vi "Scan Setup.vi"(8 "error in (no error)":errorcluster, 11 "Wavelength in":refnum<class "Wavelength Triax 550.lvclass">) -> (0 "error out":errorcluster, 3 "Wavelength out":refnum<class "Wavelength Triax 550.lvclass">)   [LabVIEW 2017, in "Wavelength Triax 550.lvclass"]
doc: "Configure the instrument based on the class member data. This step comes after the user has closed the \"Scan Setup\" window and before the actual scan -- so instruments are configured with the user's specified settings."
uses:
  Wavelength Triax 550.lvclass
  Instruments/Spectrometer Triax 550/JY-SPEX-TRIAX/controls.llb/Slits.ctl
  Wavelength Triax 550.lvclass/Wavelength Triax 550.ctl
  Scanner/Scanner.lvclass
  Instruments/Utility Classes/Scannable/Scannable.lvclass
  Instruments/Spectrometer Triax 550/JY-SPEX-TRIAX/JY-SPEX-TRIAX.lvlib
panel:
  out "User Cancelled?":bool
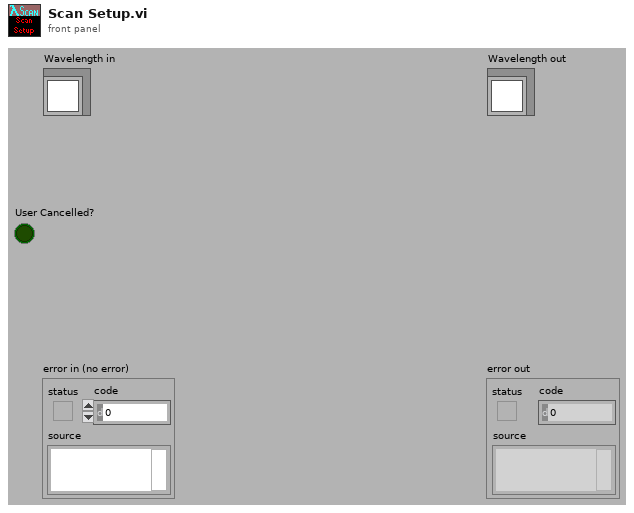
[diagram p1: front panel]
types:
  T1 = typedef "JY-SPEX-TRIAX.lvlib/Slits.ctl" = enum16{"0 (Front/Axial Entrance)", "1 (Side/Lateral Entrance)", "2 (Front/Axial Exit)", "3 (Side/Lateral Exit)"}
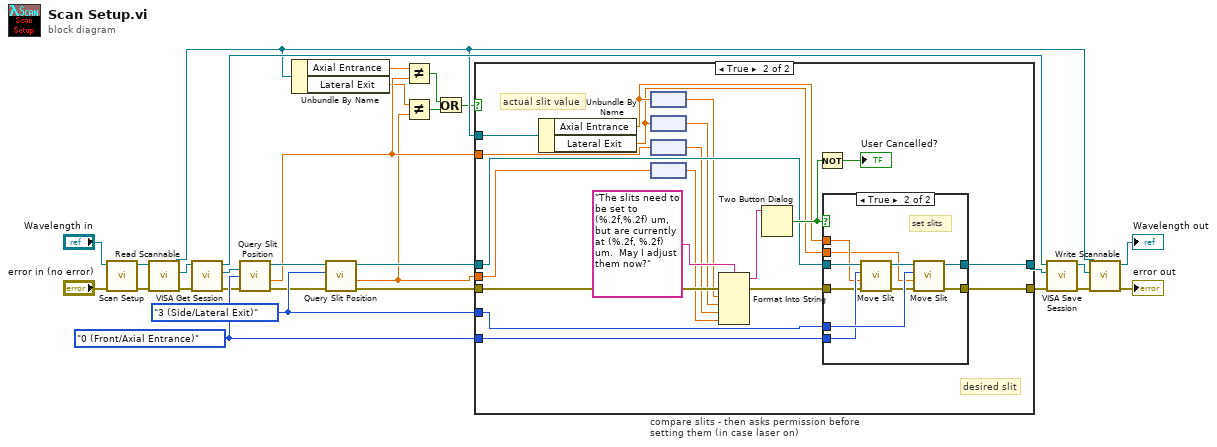
[diagram p0: block diagram]
diagram:
  w18 = Slits."3 (Side/Lateral Exit)" ("Slit (Front/Axial Entrance)")
  w17 = Slits."0 (Front/Axial Entrance)" ("Slit (Front/Axial Entrance)")
  n1 = call-parent "Scan Setup.vi"("error in (no error)"="error in (no error)", "Scanner in"="Wavelength in") -> ("error out"=w21:errorcluster, "Scanner out"=w27:refnum<class "Wavelength Triax 550.lvclass">)  [unwired: 8 out]
  n2 = call-dynamic "Read Scannable.vi"("error in (no error)"=w21, "Scanner.lvclass in"=w27) -> ("error out"=w22:errorcluster, "Scannable.lvclass"=w25:refnum<class "Scannable.lvclass">, "Scanner.lvclass out"=w7:refnum<class "Wavelength Triax 550.lvclass">)  [unwired: 7 out]
  n3 = call-dynamic "VISA Get Session.vi"("error in (no error)"=w22, "Instrument.lvclass in"=w25) -> ("error out"=w10:errorcluster, "VISA Resource Name"=w9:refnum<visa-resource-name>, "Instrument.lvclass out"=w23:refnum<class "Scannable.lvclass">)  [unwired: 7 out]
  n4 = call "Query Slit Position.vi"("error in (no error)"=w10, "Slit (Front/Axial Entrance)"=w17, "VISA resource name"=w9) -> ("error out"=w16:errorcluster, "Slit Position"=w5:dbl[unit], "VISA resource name out"=w15:refnum<visa-resource-name>)  [unwired: 1 in, 5 out]
  n5 = Unbundle By Name(w7) -> ("Axial Entrance"=w6:dbl[unit], "Lateral Exit"=w3:dbl[unit])
  n6 = call "Query Slit Position.vi"("error in (no error)"=w16, "Slit (Front/Axial Entrance)"=w18, "VISA resource name"=w15) -> ("error out"=w13:errorcluster, "Slit Position"=w2:dbl[unit], "VISA resource name out"=w14:refnum<visa-resource-name>)  [unwired: 1 in, 5 out]
  n7 = Not Equal?(x=w6, y=w5) -> (x != y?=w4:bool)
  n8 = Not Equal?(x=w3, y=w2) -> (x != y?=w8:bool)
  n9 = Or(x=w4, y=w8) -> (x .or. y?=w1:bool)
  n10 = case "compare slits - then asks permission before setting them (in case laser on)" shown="True" w1 {
    tunnel: w18 -> [_ w47]
    tunnel: w17 -> [_ w46]
    tunnel: w14 -> [w31 w45]
    tunnel: w13 -> [w30 w43]
    tunnel: [w31 w42] -> w12
    tunnel: [w30 w41] -> w11
    tunnel: w5 -> [_ w33]
    tunnel: w2 -> [_ w34]
    tunnel: w7 -> [_ w40]
    frame False {
      # "slits ok"
    }
    frame True {
      # "desired slit"
      # "actual slit value"
      n11 = Unbundle By Name(w40) -> ("Axial Entrance"=w38:dbl[unit], "Lateral Exit"=w32:dbl[unit])
      n12 = node(w38) -> (w39:dbl)
      n13 = node(w32) -> (w37:dbl)
      n14 = node(w33) -> (w36:dbl)
      n15 = node(w34) -> (w35:dbl)
      n16 = Format Into String(format string="The slits need to be set to (%.2f,%.2f) um, but are currently at (%.2f, %.2f) um.  May I adjust them now?", error in=w43, w39, w37, w36, w35) -> (resulting string=w49:string, error out=w44:errorcluster)  [unwired: 1 in]
      n17 = Two Button Dialog(message=w49) -> (T button?=w51:bool)  [unwired: 2 out]
      n18 = Not(x=w51) -> (.not. x?=→"User Cancelled?":bool)
      n19 = case shown="True" w51 {
        tunnel: w47 -> [_ w63]
        tunnel: w46 -> [_ w62]
        tunnel: w45 -> [w53 w61]
        tunnel: w44 -> [w52 w58]
        tunnel: [w53 w57] -> w42
        tunnel: [w52 w56] -> w41
        tunnel: w38 -> [_ w55]
        tunnel: w32 -> [_ w54]
        frame False {
        }
        frame True {
          # "set slits"
          n20 = call "Move Slit.vi"("error in (no error)"=w58, "Desired Slit Position"=w55, "Slit (Front/Axial Entrance)"=w62, "VISA resource name"=w61) -> ("error out"=w59:errorcluster, "VISA resource name out"=w60:refnum<visa-resource-name>)  [unwired: 1 in, 5 out]
          n21 = call "Move Slit.vi"("error in (no error)"=w59, "Desired Slit Position"=w54, "Slit (Front/Axial Entrance)"=w63, "VISA resource name"=w60) -> ("error out"=w56:errorcluster, "VISA resource name out"=w57:refnum<visa-resource-name>)  [unwired: 1 in, 5 out]
        }
      }
    }
  }
  n22 = call-dynamic "VISA Save Session.vi"("error in (no error)"=w11, "VISA Resource Name"=w12, "Instrument.lvclass in"=w23) -> ("error out"=w20:errorcluster, "Instrument.lvclass out"=w24:refnum<class "Scannable.lvclass">)  [unwired: 7 out]
  n23 = call-dynamic "Write Scannable.vi"("error in (no error)"=w20, "Scannable.lvclass"=w24, "Scanner.lvclass in"=w7) -> ("error out"=→"error out":errorcluster, "Scanner.lvclass out"=→"Wavelength out":refnum<class "Wavelength Triax 550.lvclass">)  [unwired: 7 out]
